vi "GPS-Read.vi"() -> ()   [LabVIEW 2015]
uses:
  <vilib>/Instr/_visa.llb/VISA Configure Serial Port (Instr).vi
panel:
  in  "VISA资源名称":refnum<visa-resource-name>="COM1"
  out "时间":T1
  in  "停止":bool
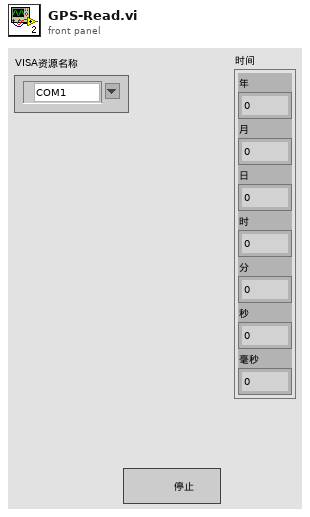
[diagram p1: front panel]
types:
  T1 = cluster{"年":u16, "月":u16, "日":u16, "时":u16, "分":u16, "秒":u16, "毫秒":u16}
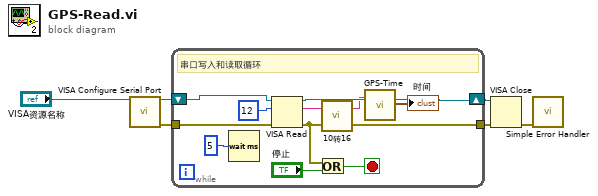
[diagram p0: block diagram]
diagram:
  n1 = call-poly "VISA Configure Serial Port"("VISA resource name"="VISA资源名称") -> ("VISA resource name out"=w2:refnum<visa-resource-name>, "error out"=w1:errorcluster)  [unwired: 9 in, 4 out]
  n2 = while {
    shift-right: [w18] -> w3
    shift-left: w2 -> [w14]
    tunnel: [w9] -> w4
    tunnel: w1 -> [w11]
    stop <- w16 stop-if-true
    # "串口写入和读取循环"
    n3 = Wait (ms)(milliseconds to wait=u32 5) -> ()  [unwired: 1 out]
    n4 = VISA Read(VISA resource name=w14, byte count=u32 12 ("Bytes at Port"), error in (no error)=w11) -> (VISA resource name out=w18:refnum<visa-resource-name>, read buffer=w12:string, error out=w10:errorcluster)  [unwired: 1 out]
    n5 = Or(x=w10, y="停止") -> (x .or. y?=w16:bool)
    n6 = call "10转16.vi"("错误In"=w10, "字符串"=w12) -> ("错误Out"=w9:errorcluster, "字符串 2"=w7:string)
    n7 = call "GPS-Time.vi"("响应"=w7) -> ("时间"=→"时间":T1)  [unwired: 1 in, 1 out]
  }
  n8 = VISA Close(VISA resource name=w3, error in (no error)=w4) -> (error out=w5:errorcluster)
  n9 = call <vilib>:"Simple Error Handler.vi"("error in (no error)"=w5) -> ()  [unwired: 1 in, 8 out]
